vi "Diode-Trace-Data.vi"(0 "connection ID":refnum<k5>, 11 "error in (no error)":errorcluster) -> (2 "ymin":dbl, 3 "ymax":dbl, 4 "connection ID out":refnum<k5>, 6 "Trace (Raw ADC)":u16[](array[numeric]), 8 "Trace (Volts)":dbl[](array[numeric]), 10 "dt":dbl, 13 "Background Mask Array":bool[](array[boolean]), 14 "Signal Mask Array":bool[](array[boolean]), 15 "error out":errorcluster)   [LabVIEW 2020]
panel:
  out "T1 (secs)":dbl
  out "T4-NT":i32
  out "T3-NT":i32
  out "NT":i32
  out "T2-NT":i32
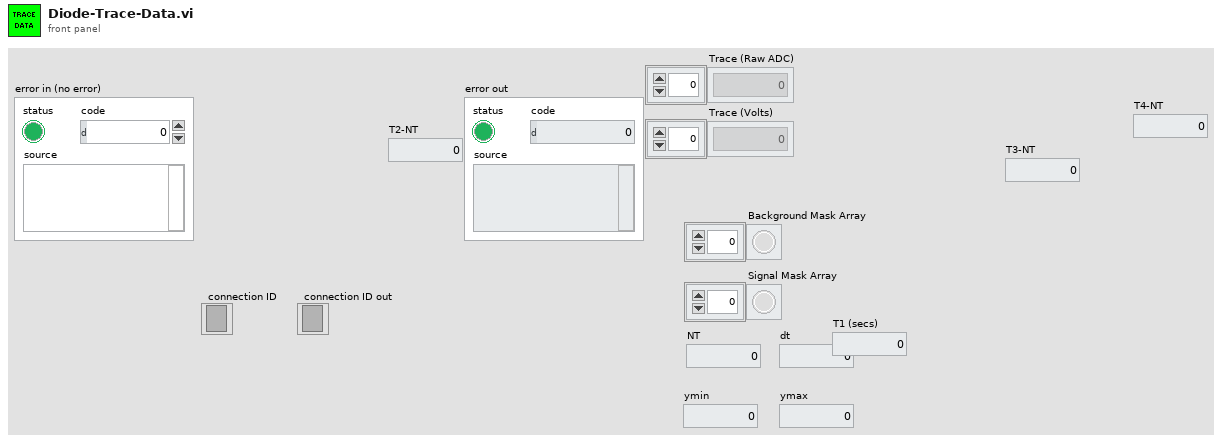
[diagram p1: front panel]
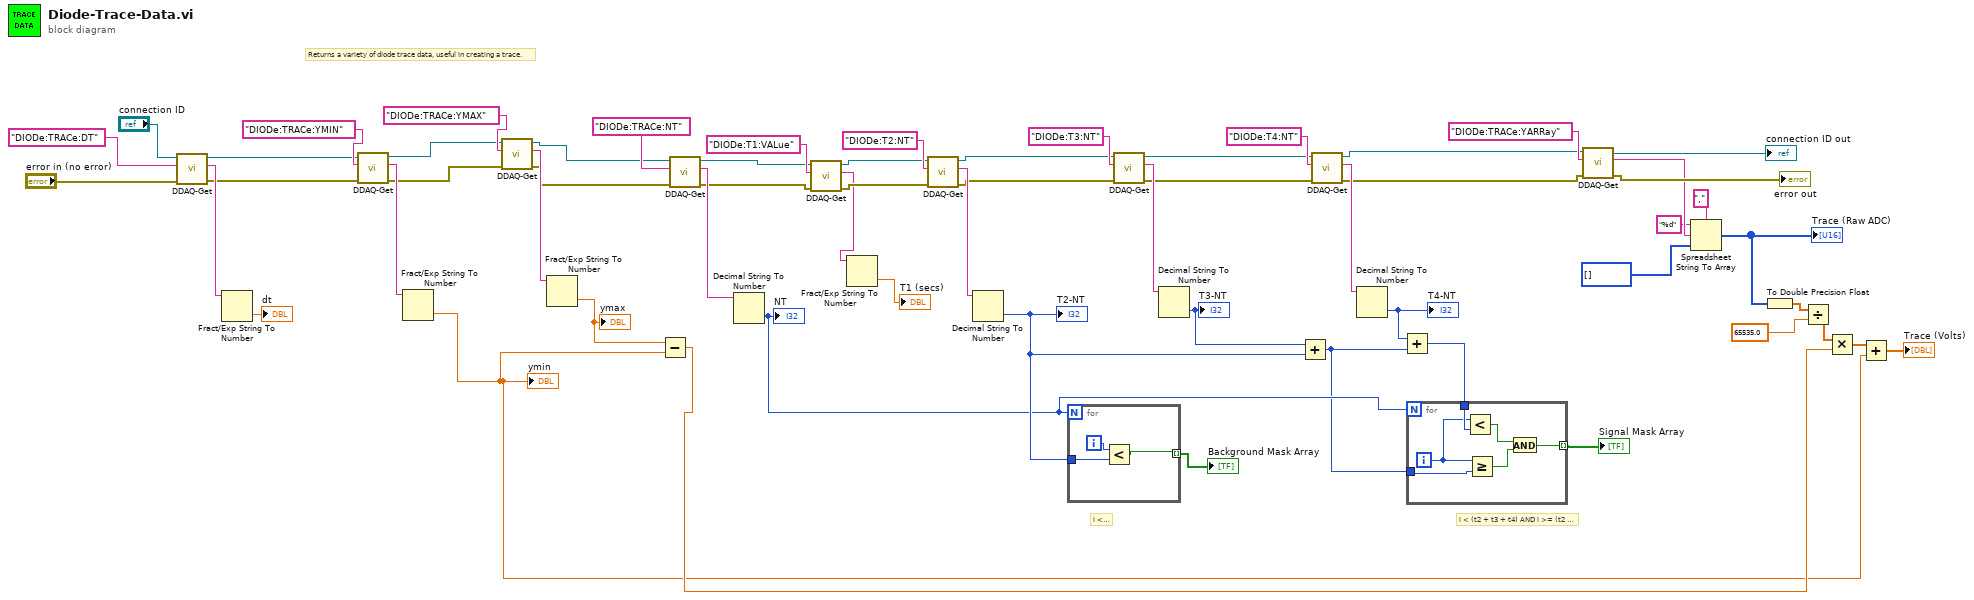
[diagram p0: block diagram]
diagram:
  # "i < (t2 + t3 + t4) AND i >= (t2 + t3)"
  # "i < t2"
  # "Returns a variety of diode trace data, useful in creating a trace."
  n1 = call "DDAQ-Get.vi"("error in (no error)"="error in (no error)", "SCPI-like Keyword (leave off question mark)"="DIODe:TRACe:DT" ("Diode Keyword (leave off question mark)"), "connection ID"="connection ID") -> ("error out"=w41:errorcluster, "Response"=w60:string, "connection ID out"=w42:refnum<k5>)  [unwired: 5 in, 1 out]
  n2 = Fract/Exp String To Number(string=w60) -> (number=→"dt":dbl)  [unwired: 3 in, 1 out]
  n3 = call "DDAQ-Get.vi"("error in (no error)"=w41, "SCPI-like Keyword (leave off question mark)"="DIODe:TRACe:YMIN" ("Diode Keyword (leave off question mark)"), "connection ID"=w42) -> ("error out"=w37:errorcluster, "Response"=w44:string, "connection ID out"=w38:refnum<k5>)  [unwired: 5 in, 1 out]
  n4 = Fract/Exp String To Number(string=w44) -> (number=w9:dbl)  [unwired: 3 in, 1 out]
  "ymin" <- w9
  n5 = call "DDAQ-Get.vi"("error in (no error)"=w37, "SCPI-like Keyword (leave off question mark)"="DIODe:TRACe:YMAX" ("Diode Keyword (leave off question mark)"), "connection ID"=w38) -> ("error out"=w36:errorcluster, "Response"=w40:string, "connection ID out"=w35:refnum<k5>)  [unwired: 5 in, 1 out]
  n6 = Fract/Exp String To Number(string=w40) -> (number=w15:dbl)  [unwired: 3 in, 1 out]
  "ymax" <- w15
  n7 = Subtract(x=w15, y=w9) -> (x-y=w11:dbl)
  n8 = call "DDAQ-Get.vi"("error in (no error)"=w36, "SCPI-like Keyword (leave off question mark)"="DIODe:TRACe:NT" ("Diode Keyword (leave off question mark)"), "connection ID"=w35) -> ("error out"=w5:errorcluster, "Response"=w54:string, "connection ID out"=w6:refnum<k5>)  [unwired: 5 in, 1 out]
  n9 = Decimal String To Number(string=w54) -> (number=w31:i32)  [unwired: 2 in, 1 out]
  "NT" <- w31
  n10 = call "DDAQ-Get.vi"("error in (no error)"=w5, "SCPI-like Keyword (leave off question mark)"="DIODe:T1:VALue" ("Diode Keyword (leave off question mark)"), "connection ID"=w6) -> ("error out"=w4:errorcluster, "Response"=w1:string, "connection ID out"=w3:refnum<k5>)  [unwired: 5 in, 1 out]
  n11 = Fract/Exp String To Number(string=w1) -> (number=→"T1 (secs)":dbl)  [unwired: 3 in, 1 out]
  n12 = call "DDAQ-Get.vi"("error in (no error)"=w4, "SCPI-like Keyword (leave off question mark)"="DIODe:T2:NT" ("Diode Keyword (leave off question mark)"), "connection ID"=w3) -> ("error out"=w47:errorcluster, "Response"=w56:string, "connection ID out"=w48:refnum<k5>)  [unwired: 5 in, 1 out]
  n13 = Decimal String To Number(string=w56) -> (number=w32:i32)  [unwired: 2 in, 1 out]
  "T2-NT" <- w32
  n14 = for {
    N: w31 -> [_]
    tunnel: [w63] -> w34 mode=indexing
    tunnel: w32 -> [w61]
    i -> [w62]
    n15 = Less?(x=w62, y=w61) -> (x < y?=w63:bool)
  }
  "Background Mask Array" <- w34
  n16 = call "DDAQ-Get.vi"("error in (no error)"=w47, "SCPI-like Keyword (leave off question mark)"="DIODe:T3:NT" ("Diode Keyword (leave off question mark)"), "connection ID"=w48) -> ("error out"=w46:errorcluster, "Response"=w52:string, "connection ID out"=w49:refnum<k5>)  [unwired: 5 in, 1 out]
  n17 = Decimal String To Number(string=w52) -> (number=w33:i32)  [unwired: 2 in, 1 out]
  "T3-NT" <- w33
  n18 = Add(x=w33, y=w32) -> (x+y=w28:i32)
  n19 = call "DDAQ-Get.vi"("error in (no error)"=w46, "SCPI-like Keyword (leave off question mark)"="DIODe:T4:NT" ("Diode Keyword (leave off question mark)"), "connection ID"=w49) -> ("error out"=w23:errorcluster, "Response"=w50:string, "connection ID out"=w24:refnum<k5>)  [unwired: 5 in, 1 out]
  n20 = Decimal String To Number(string=w50) -> (number=w30:i32)  [unwired: 2 in, 1 out]
  "T4-NT" <- w30
  n21 = Add(x=w30, y=w28) -> (x+y=w29:i32)
  n22 = for {
    N: w31 -> [_]
    tunnel: w29 -> [w69]
    tunnel: w28 -> [w66]
    tunnel: [w64] -> w27 mode=indexing
    i -> [w67]
    n23 = Less?(x=w67, y=w69) -> (x < y?=w68:bool)
    n24 = Greater Or Equal?(x=w67, y=w66) -> (x >= y?=w65:bool)
    n25 = And(x=w68, y=w65) -> (x .and. y?=w64:bool)
  }
  "Signal Mask Array" <- w27
  n26 = call "DDAQ-Get.vi"("error in (no error)"=w23, "SCPI-like Keyword (leave off question mark)"="DIODe:TRACe:YARRay" ("Diode Keyword (leave off question mark)"), "connection ID"=w24) -> ("error out"=→"error out":errorcluster, "Response"=w20:string, "connection ID out"=→"connection ID out":refnum<k5>)  [unwired: 5 in, 1 out]
  n27 = Spreadsheet String To Array(delimiter (Tab)=",", format string="%d", spreadsheet string=w20, array type (2D Dbl)=u16[] []) -> (array=w16:u16[])
  "Trace (Raw ADC)" <- w16
  n28 = To Double Precision Float(number=w16) -> (double precision float=w14:dbl[])
  n29 = Divide(x=w14, y=65535.0) -> (x/y=w12:dbl[])
  n30 = Multiply(x=w12, y=w11) -> (x*y=w10:dbl[])
  n31 = Add(x=w10, y=w9) -> (x+y=→"Trace (Volts)":dbl[])
